vi "Init.vi"(8 "error in (no error)":errorcluster, 10 "HTTP Server":refnum<class "Server.lvclass">) -> (0 "error out":errorcluster, 3 "HTTPServerService out":refnum<class "HTTPServerService.lvclass">)   [LabVIEW 2020, in "Vecto.lvlib" / "HTTPServerService.lvclass"]
uses:
  HTTPServerService.lvclass
  <vilib>/IlluminatedG/IG HTTP Server/HTTP Server/Server/Server.lvclass
  HTTPServerService.lvclass/HTTPServerService.ctl
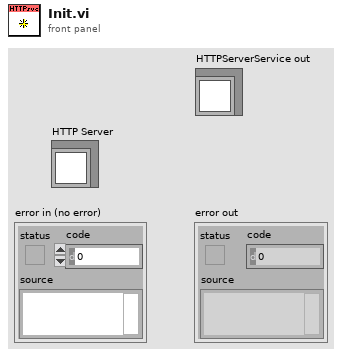
[diagram p1: front panel]
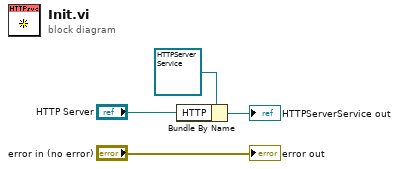
[diagram p0: block diagram]
diagram:
  n1 = Bundle By Name(cluster=refnum<class "HTTPServerService.lvclass"> refnum ("HTTPServerService in"), "HTTP"="HTTP Server") -> (→"HTTPServerService out":refnum<class "HTTPServerService.lvclass">)
  "error out" <- "error in (no error)"
